vi "test harness_FXP_A_times_x_iterate.vi"() -> ()   [LabVIEW 2017, in "FXP_observer_TestCase.lvclass"]
uses:
  FXP_observer_TestCase.lvclass
  fpga_VIs/fpga_subVIs_ssxy/fixed-point-ss/typeDefs/x_vec_scalar.ctl
  <vilib>/rvi/DesktopExecutionNode/Execution/niFpgaDEN_Execute.vi
  <vilib>/rvi/DesktopExecutionNode/DesktopExecutionNode.xnode
panel:
  out "error out":errorcluster
  out "TestCase out":refnum<class "FXP_observer_TestCase.lvclass">
  in  "TestCase in":refnum<class "FXP_observer_TestCase.lvclass">
  in  "error in (no error)":errorcluster
  out "X_vec":T1[](array[typedef])
  out "xk_1_1":fxp<+/-,32,6>[](array[numeric])
  out "A*x":fxp<+/-,32,13>[](array[numeric])
  out "y(exp)":fxp<+/-,64,17>
  out "A*x (expected)":fxp<+/-,64,12>[](array[numeric])
  out "Waveform Graph":dbl[](graph)
  out "Y":fxp<+/-,32,6>[](array[numeric])
  in  "NumIter":i32=1
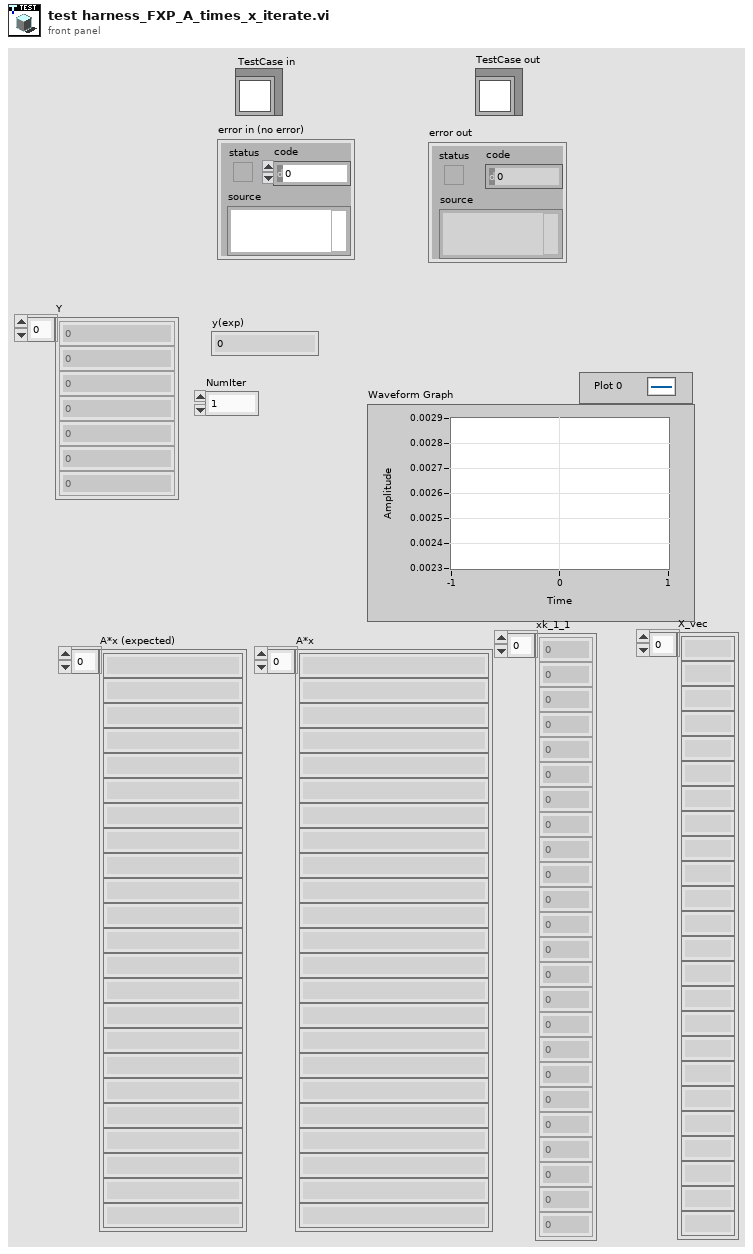
[diagram p1: front panel]
types:
  T1 = typedef "x_vec_scalar.ctl" = fxp<+/-,32,6>
  T2 = typedef "UT_matrix_data.ctl" = cluster{"Bz":T3[], "Ldist":T4[], "Kz":T5[], "Nx":T6[], "Ax_col":T7[], "X_vec":T1[], "Cz":T8[]}
  T3 = typedef "Bz_vec_scalar.ctl" = fxp<+/-,32,3>
  T4 = typedef "Lz_vec_scalar.ctl" = fxp<+/-,32,3>
  T5 = typedef "Kz_vec_scalar.ctl" = fxp<+/-,32,10>
  T6 = typedef "Nx_vec_scalar.ctl" = fxp<+/-,32,2>
  T7 = typedef "Az_vec_scalar.ctl" = fxp<+/-,32,7>
  T8 = typedef "Cz_vec_scalar.ctl" = fxp<+/-,32,4>
  T9 = typedef "x_vec_type.ctl" = fxp<+/-,32,6>[]
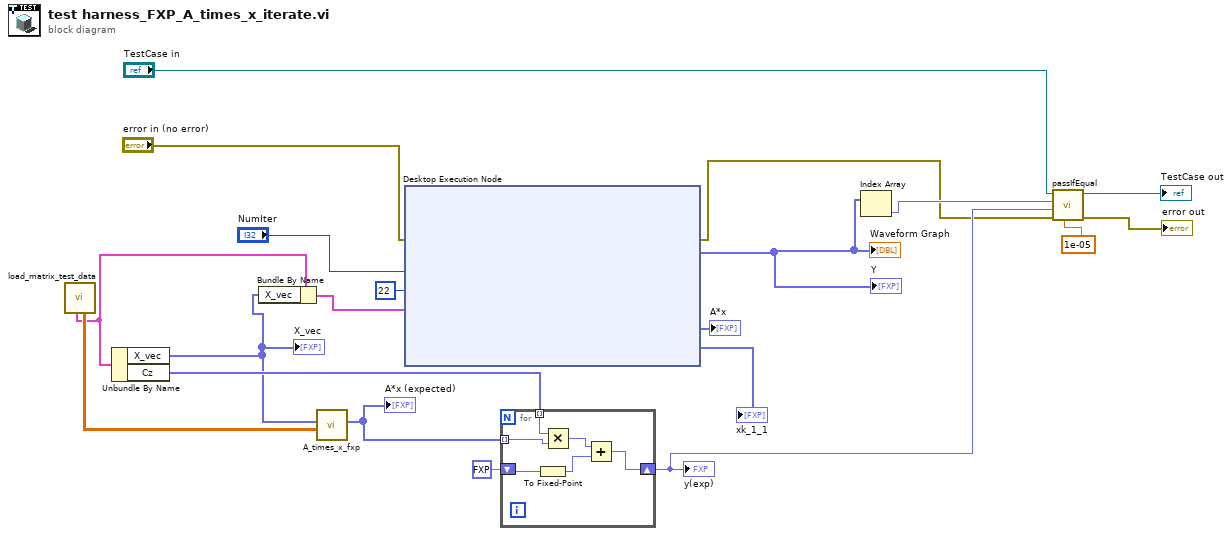
[diagram p0: block diagram]
diagram:
  n1 = call "load_matrix_test_data.vi"() -> ("A_mat"=w18:dbl[][], "output cluster"=w12:T2)  [unwired: 4 in, 6 out]
  n2 = Unbundle By Name(w12) -> ("X_vec"=w11:T1[], "Cz"=w16:T8[])
  "X_vec" <- w11
  n3 = Bundle By Name(cluster=w12, "X_vec"=w11) -> (w10:T2)
  n4 = call "A_times_x_fxp.vi"("Az_mat in"=w18, "x_vec"=w11) -> ("A*x"=w17:T9)  [unwired: 8 in, 1 out]
  "A*x (expected)" <- w17
  n5 = xnode "Desktop Execution Node"("Error In"="error in (no error)", "NumIter"="NumIter", "NS"=u8 22 ("NS + 1"), "matrix data"=w10) -> ("Error Out"=w3:errorcluster, "Y"=w8:fxp<+/-,32,6>[], "A*x"=→"A*x":fxp<+/-,32,13>[], "xk_1_1"=→"xk_1_1":fxp<+/-,32,6>[])
  "Y" <- w8
  "Waveform Graph" <- w8
  n6 = for {
    tunnel: w17 -> [w25] mode=indexing
    tunnel: w16 -> [w26] mode=indexing
    shift-right: [w23] -> w7
    shift-left: fxp<+/-,64,17> 0.0 -> [w21]
    n7 = To Fixed-Point(number=w21) -> (fixed-point=w22:fxp<+/-,64,13>)  [unwired: 1 in]
    n8 = Multiply(x=w26, y=w25) -> (x*y=w24:fxp<+/-,64,10>)
    n9 = Add(x=w24, y=w22) -> (x+y=w23:fxp<+/-,64,14>)
  }
  "y(exp)" <- w7
  n10 = Index Array(array=w8) -> (element=w6:fxp<+/-,32,6>)  [unwired: 1 in]
  n11 = call-dynamic "passIfEqual.vi"("delta (optional)"=1e-05, "error in (no error)"=w3, "y"=w7, "x"=w6, "TestCase in"="TestCase in") -> ("error out"=→"error out":errorcluster, "TestCase out"=→"TestCase out":refnum<class "FXP_observer_TestCase.lvclass">)  [unwired: 5 in]
